vi "get column types.vi"(8 "error in (no error)":errorcluster, 11 "active statement":T1={"ppStmt"=0, "column count"=0, "bind offset"=1, "bind param count"=1, "finished?"=FALSE, "column offset"=0, "column types"=[]} {"column types" items=["INTEGER"=1, "FLOAT"=2, "STRING"=3, "BLOB"=4, "NULL"=5]}) -> (0 "error out":errorcluster, 3 "column types out":i32[](array[ring]) items=["INTEGER"=1, "FLOAT"=2, "STRING"=3, "BLOB"=4, "NULL"=5])   [LabVIEW 2014, in "SQLite3LV.lvlib" / "cursor.lvclass"]
uses:
  cursor.lvclass
  ctl_active_statement.ctl
  sqlite3_64.dll
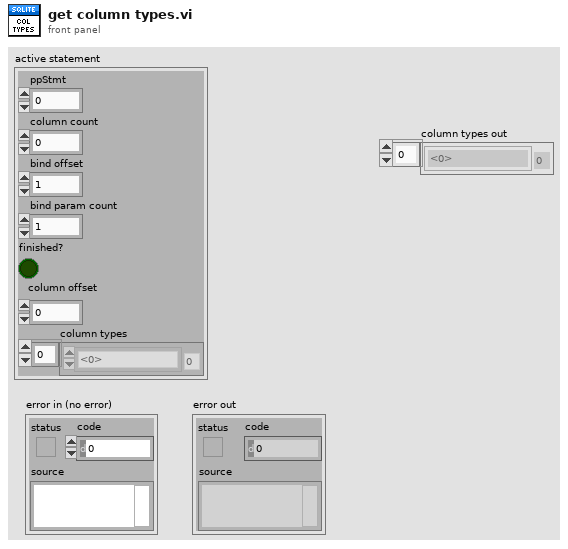
[diagram p1: front panel]
types:
  T1 = typedef "SQLite3LV.lvlib/cursor.lvclass/ctl_active_statement.ctl" = cluster{"ppStmt":i64, "column count":i32, "bind offset":i32, "bind param count":i32, "finished?":bool, "column offset":i32, "column types":i32[]}
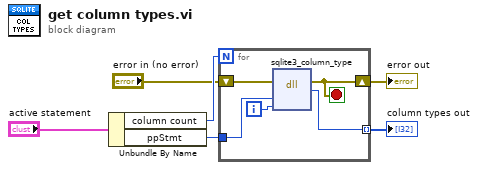
[diagram p0: block diagram]
diagram:
  n1 = Unbundle By Name("active statement") -> ("column count"=w3:i32, "ppStmt"=w4:i64)
  n2 = for {
    N: w3 -> [_]
    tunnel: w4 -> [w11]
    tunnel: [w9] -> w5 mode=indexing
    shift-right: [w7] -> w1
    shift-left: "error in (no error)" -> [w8]
    i -> [w10]
    stop <- w7 stop-if-true
    n3 = dll-call lib="C:/Users/BobUser/Desktop/LVTables/sqlite3**.*" fn="sqlite3_column_type"(error in=w8, "pStmt"=w11, "iCol"=w10) -> (error out=w7:errorcluster, "column type"=w9:i32)  [unwired: 4 in, 1 out]
  }
  "column types out" <- w5
  "error out" <- w1
